vi "OP500Z8P_ITECH_CONF.vi"(8 "ErrIN":errorcluster caption="errin", 11 "VISAin":refnum<visa-resource-name>) -> (0 "ErrOUT":errorcluster caption="errout", 3 "VisaOUT":refnum<visa-resource-name>)   [LabVIEW 2020]
uses:
  <instrlib>/IT6000C/IT6000C.lvlib
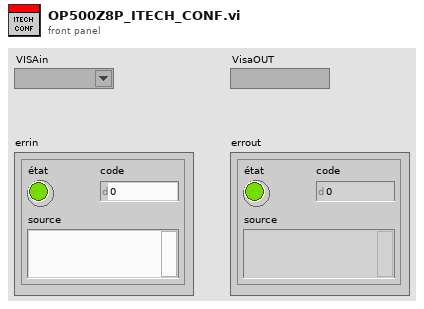
[diagram p1: front panel]
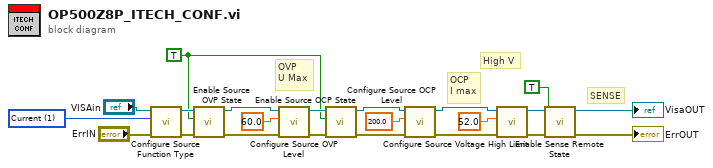
[diagram p0: block diagram]
diagram:
  w12 = u16 1 items=["Voltage", "Current"] ("Mode(0:Voltage)")
  w2 = TRUE ("Enable(True)")
  # "High V"
  # "SENSE"
  # "OVP\nU Max"
  # "OCP\nI max"
  n1 = call <instrlib>:"Configure Source Function Type.vi"("error in (no error)"="ErrIN", "Mode(0:Voltage)"=w12, "VISA resource name"="VISAin") -> ("error out"=w10:errorcluster, "VISA resource name out"=w11:refnum<visa-resource-name>)  [unwired: 7 in]
  n2 = call <instrlib>:"Enable Source OVP State.vi"("error in (no error)"=w10, "Enable(True)"=w2, "VISA resource name"=w11) -> ("error out"=w20:errorcluster, "VISA resource name out"=w19:refnum<visa-resource-name>)  [unwired: 7 in]
  n3 = call <instrlib>:"Configure Source OVP Level.vi"("error in (no error)"=w20, "Value(0)"=60.0, "VISA resource name"=w19) -> ("error out"=w18:errorcluster, "VISA resource name out"=w17:refnum<visa-resource-name>)  [unwired: 7 in]
  n4 = call <instrlib>:"Enable Source OCP State.vi"("error in (no error)"=w18, "Enable(True)"=w2, "VISA resource name"=w17) -> ("error out"=w15:errorcluster, "VISA resource name out"=w16:refnum<visa-resource-name>)  [unwired: 7 in]
  n5 = call <instrlib>:"Configure Source OCP Level.vi"("error in (no error)"=w15, "Value(0)"=200.0, "VISA resource name"=w16) -> ("error out"=w9:errorcluster, "VISA resource name out"=w8:refnum<visa-resource-name>)  [unwired: 7 in]
  n6 = call <instrlib>:"Configure Source Voltage High Limit.vi"("error in (no error)"=w9, "Value(0)"=52.0, "VISA resource name"=w8) -> ("error out"=w6:errorcluster, "VISA resource name out"=w5:refnum<visa-resource-name>)  [unwired: 7 in]
  n7 = call <instrlib>:"Enable Sense Remote State.vi"("error in (no error)"=w6, "Enable(True)"=TRUE, "VISA resource name"=w5) -> ("error out"=→"ErrOUT":errorcluster, "VISA resource name out"=→"VisaOUT":refnum<visa-resource-name>)  [unwired: 7 in]
